vi "utilities_binaryFileCreate.vi"(8 "error in (no error)":errorcluster, 11 "path":path) -> (0 "error out":errorcluster, 3 "refnum out":refnum<k1>)   [LabVIEW 2020, in "NI_ExcelFile.lvlib"]
uses:
  <vilib>/express/express shared/NI_ExcelFile/NI_ExcelFile.lvlib
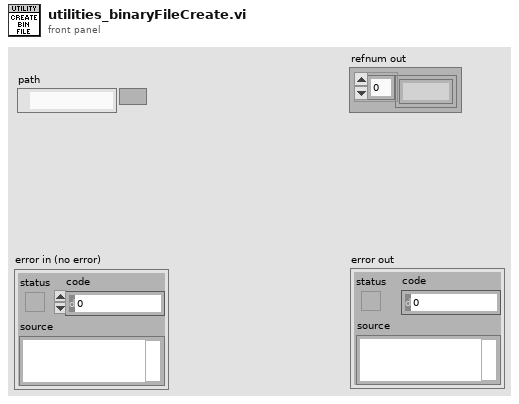
[diagram p1: front panel]
types:
  T1 = enum16{"open", "replace", "create", "open or create", "replace or create", "replace or create with confirmation"}
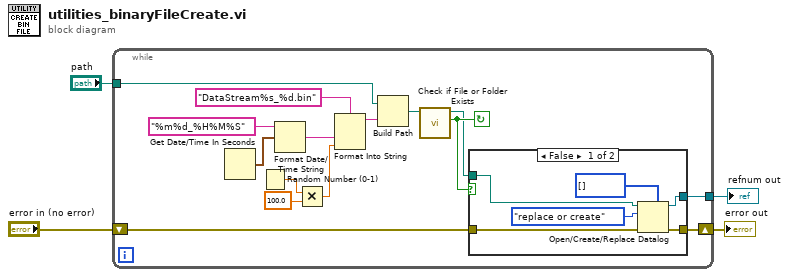
[diagram p0: block diagram]
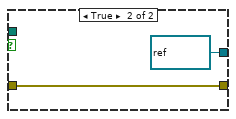
[diagram p2: hidden frame]
diagram:
  n1 = while {
    tunnel: "path" -> [w19]
    shift-right: [w6] -> w4
    shift-left: "error in (no error)" -> [w7]
    tunnel: [w5] -> w1
    stop <- w9 continue-if-true
    n2 = Get Date/Time In Seconds() -> (seconds since 1Jan1904=w16:timestamp)
    n3 = Random Number (0-1)() -> (number: 0 to 1=w13:dbl)
    n4 = Format Date/Time String(time format string (%c)="%m%d_%H%M%S", seconds (now)=w16) -> (date/time string=w14:string)  [unwired: 1 in]
    n5 = Multiply(x=w13, y=100.0) -> (x*y=w11:dbl)
    n6 = Format Into String(format string="DataStream%s_%d.bin" ("name or relative path"), w14, w11) -> (resulting string=w17:string)  [unwired: 2 in, 1 out]
    n7 = Build Path(base path=w19, name or relative path=w17) -> (appended path=w10:path)
    n8 = call <vilib>:"Check if File or Folder Exists.vi"("path"=w10) -> ("file or folder exists?"=w9:bool, "dup path"=w8:path)  [unwired: 8 in, 1 out]
    n9 = case shown="False" w9 {
      tunnel: w8 -> [w24 _]
      tunnel: w7 -> [w22 w27]
      tunnel: [w21 w27] -> w6
      tunnel: [w20 refnum<k1> refnum] -> w5
      frame False {
        n10 = Open/Create/Replace Datalog(5:u8[] [], 8:w22, 10:T1."replace or create" ("operation (0:open)"), 11:w24) -> (0:w21:errorcluster, 3:w20:refnum<k1>)  [unwired: 2 in, 1 out]
      }
      frame True {
      }
    }
  }
  "error out" <- w4
  "refnum out" <- w1
